vi "SSCP.vi"(0 "Config file path":path=path "F:/Projects/simple-system-control-protocol/simple-system-control-protocol/source/python/lp_em_cc2340r5_example.yml", 1 "Parameter name":string, 2 "Parameter value":string, 3 "Register name":string, 5 "Device Configuration":T1={"Device name"="default", "Device number"="0", "Serial Port"="COM9", "Serial baud rate"="115200", "Base Port"="3000", "Device Serial Number"="1", "Interface Timeout"="10000", "Interface Type"="SERIAL"}, 11 "error in (no error)":errorcluster, 12 "Command":T2) -> (4 "Parameter value":dbl, 15 "error out":errorcluster)   [LabVIEW 2020]
uses:
  commands.ctl
  typedefs/Device Configuration.ctl
  typedefs/Parameter Descriptor.ctl
  typedefs/Register Descriptor.ctl
  <vilib>/regexp/Match Regular Expression.xnode
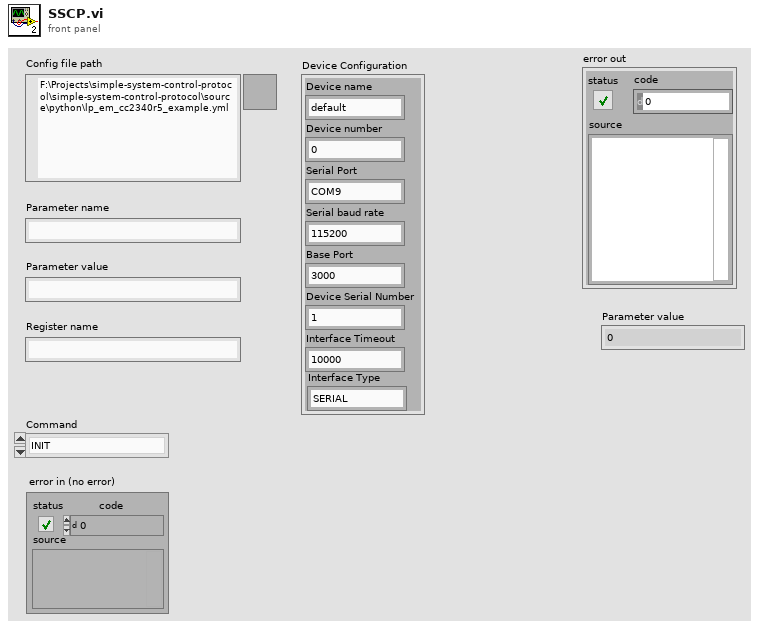
[diagram p1: front panel]
types:
  T1 = typedef "Device Configuration.ctl" = cluster{"Device name":string, "Device number":string, "Serial Port":string, "Serial baud rate":string, "Base Port":string, "Device Serial Number":string, "Interface Timeout":string, "Interface Type":string}
  T2 = typedef "commands.ctl" = enum16{"INIT", "CONFIGURE", "CONNECT", "GET_PARAMETER", "GET_PARAMETER_FROM_DEVICE", "SET_PARAMETER", "SET_PARAMETER_IN_DEVICE", "READ_REGISTER", "WRITE_REGISTER", "DISCONNECT"}
  T3 = typedef "Register Descriptor.ctl" = cluster{"Parameter Descriptors":T4[], "Register name":string, "Register number":i32}
  T4 = typedef "Parameter Descriptor.ctl" = cluster{"Register name":string, "Parameter name":string, "Register number":i32, "Parameter number":i32, "Start Bit":i32, "Bit Length":i32, "min":string, "max":string, "datatype":string}
  T5 = enum16{"Standard", "Buffered", "CRLF", "Immediate"}
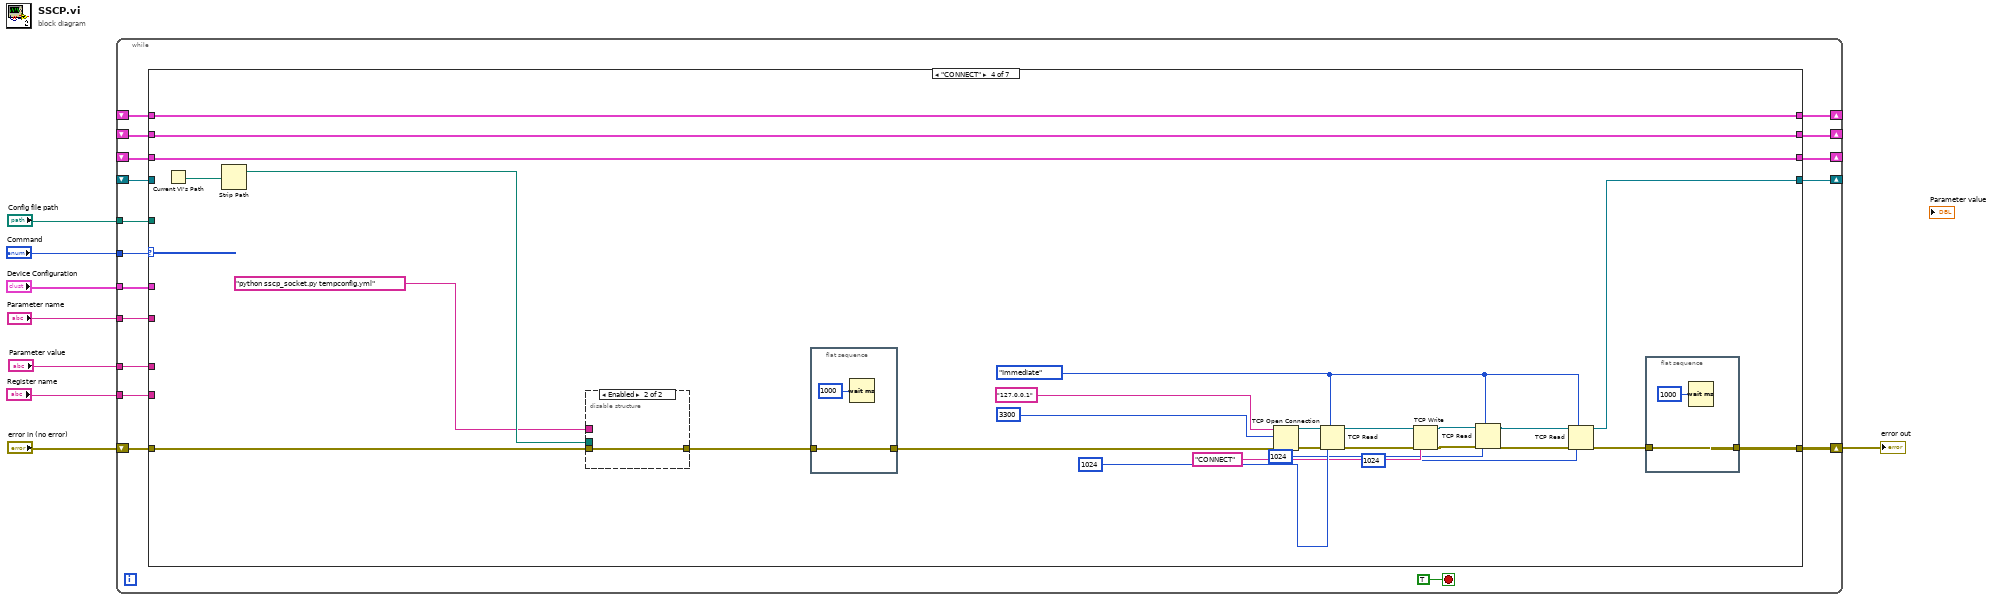
[diagram p0: block diagram]
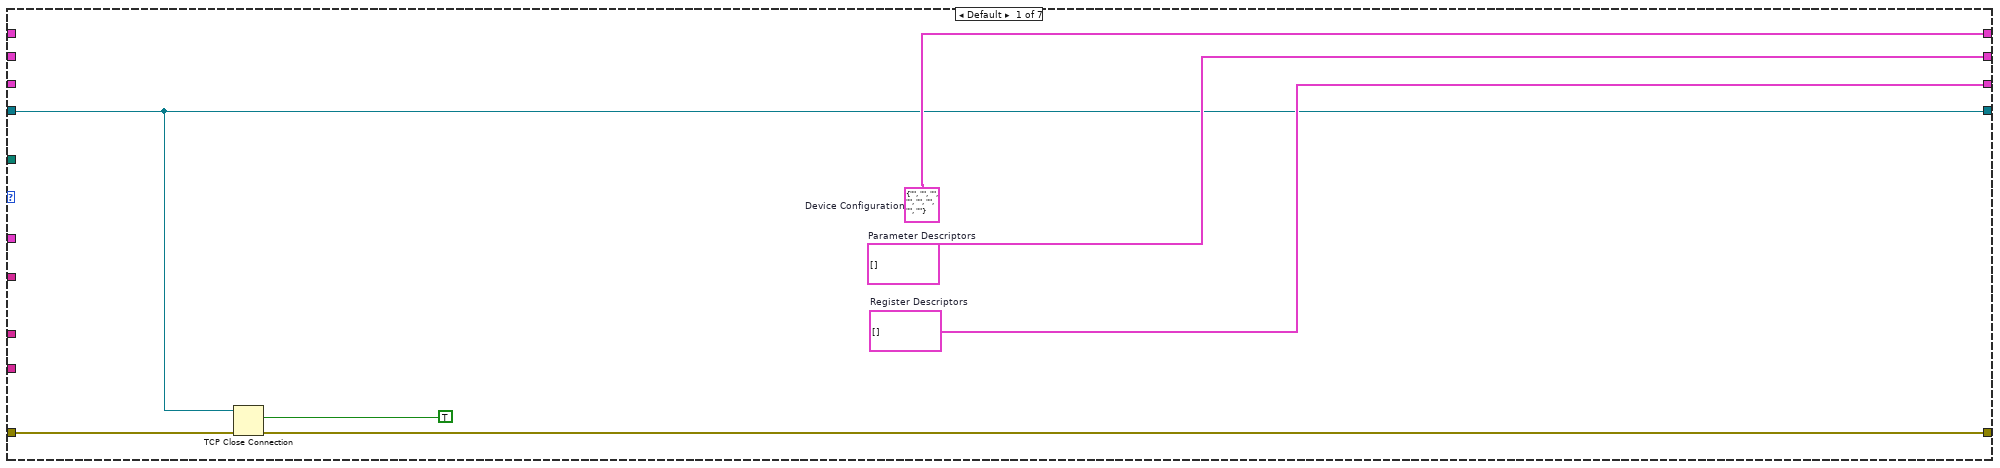
[diagram p2: hidden frame]
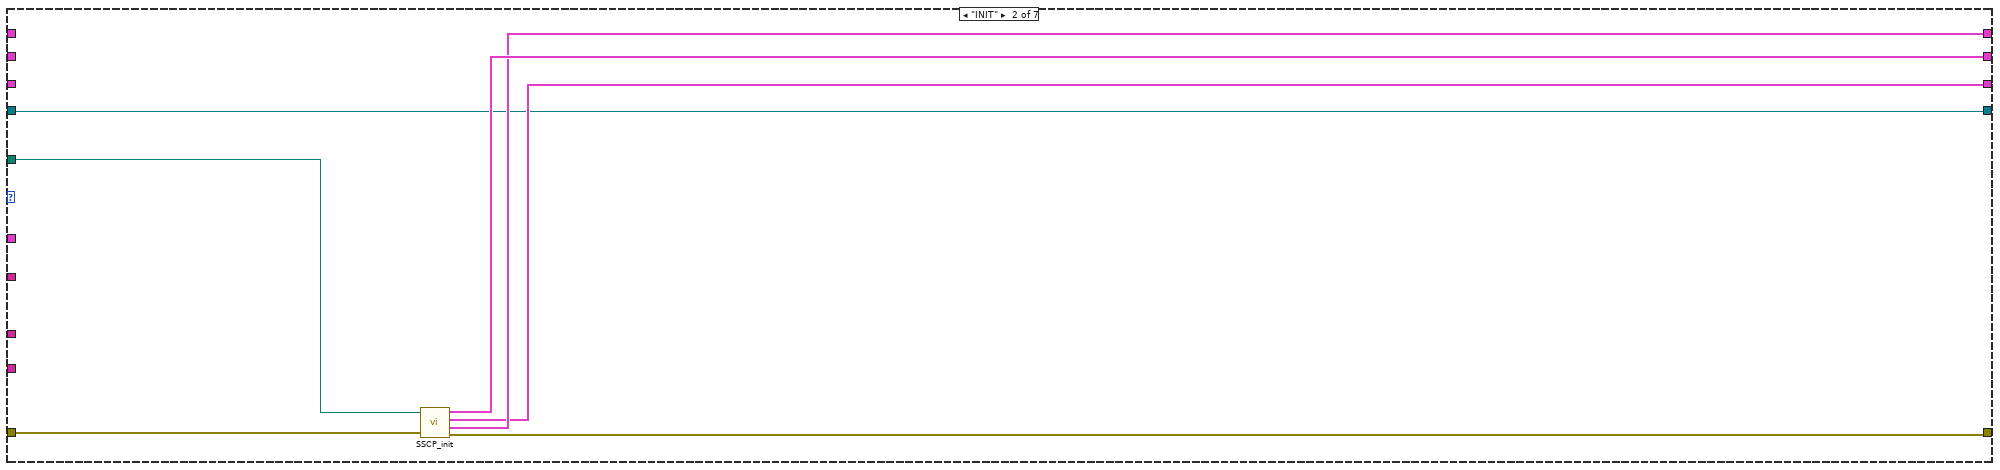
[diagram p3: hidden frame]
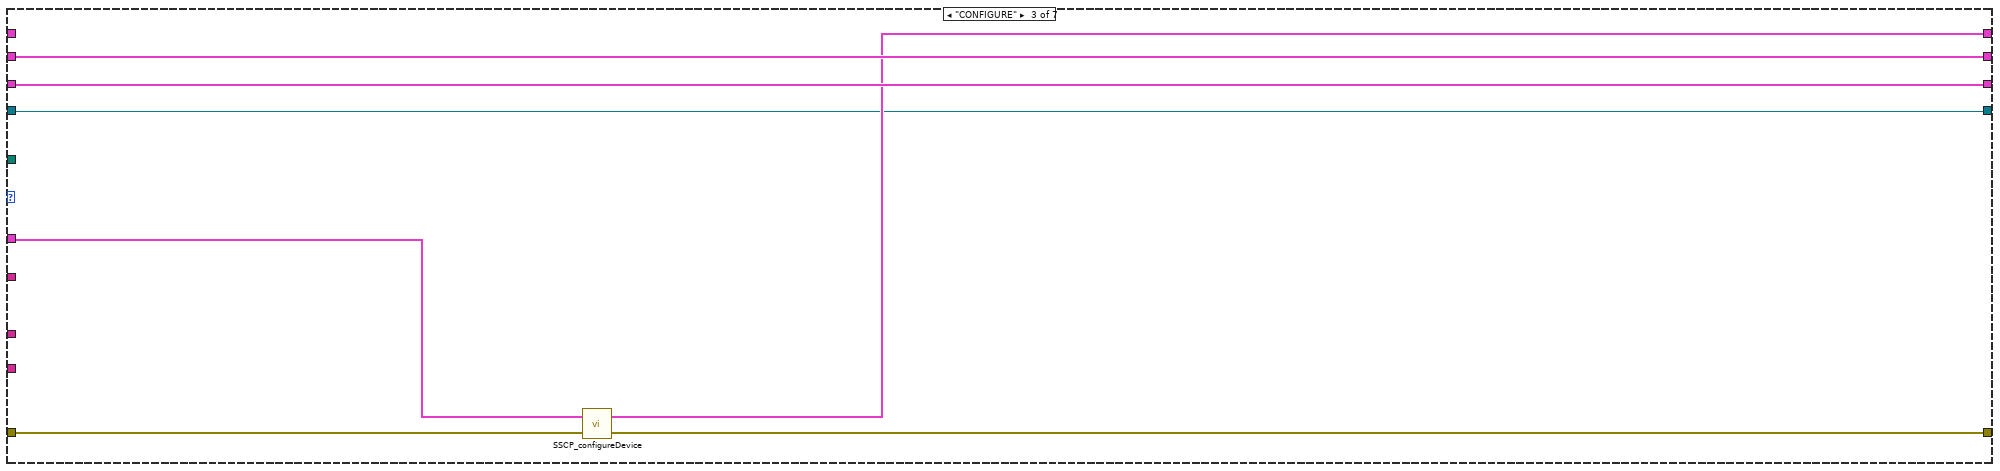
[diagram p4: hidden frame]
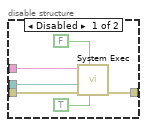
[diagram p5: hidden frame]
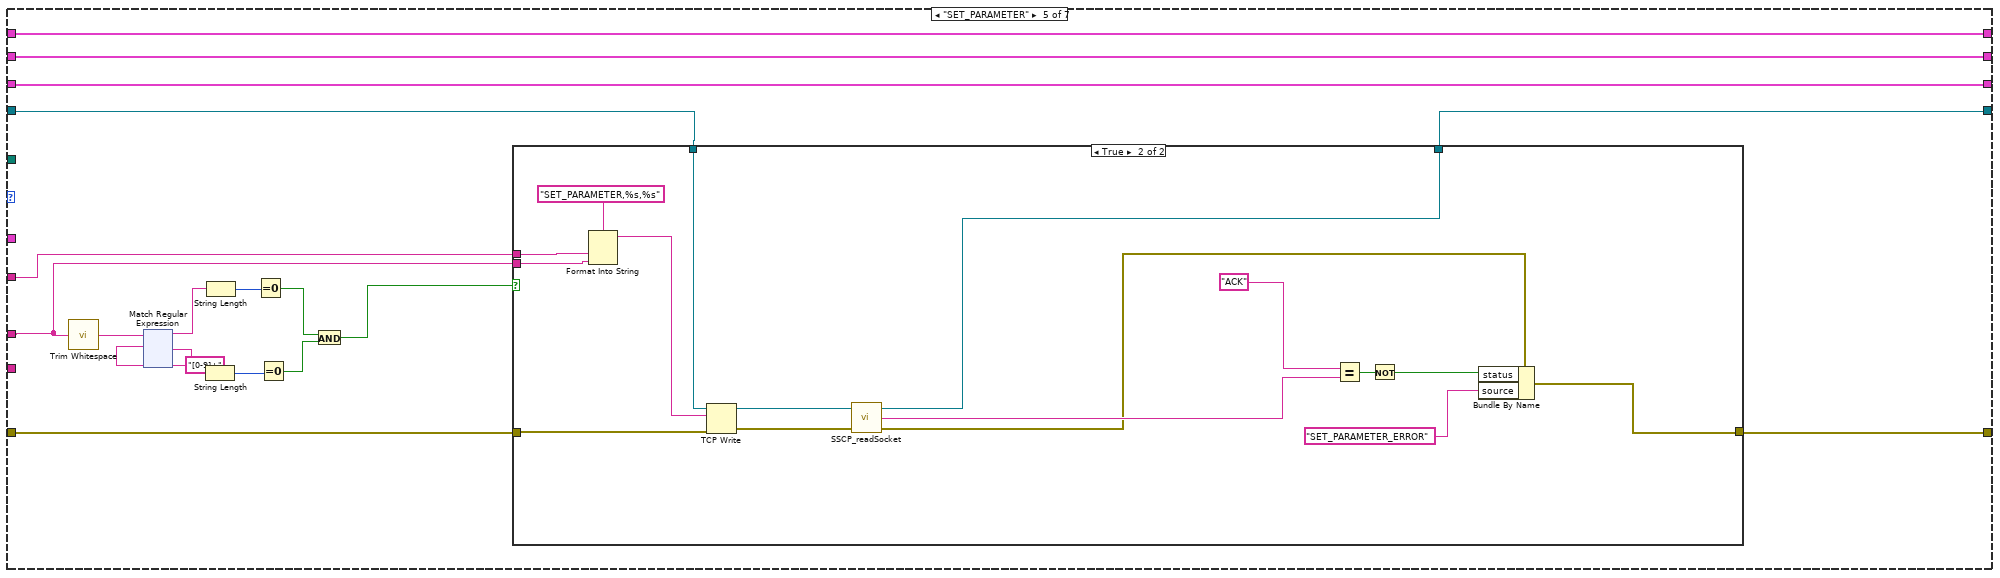
[diagram p6: hidden frame]
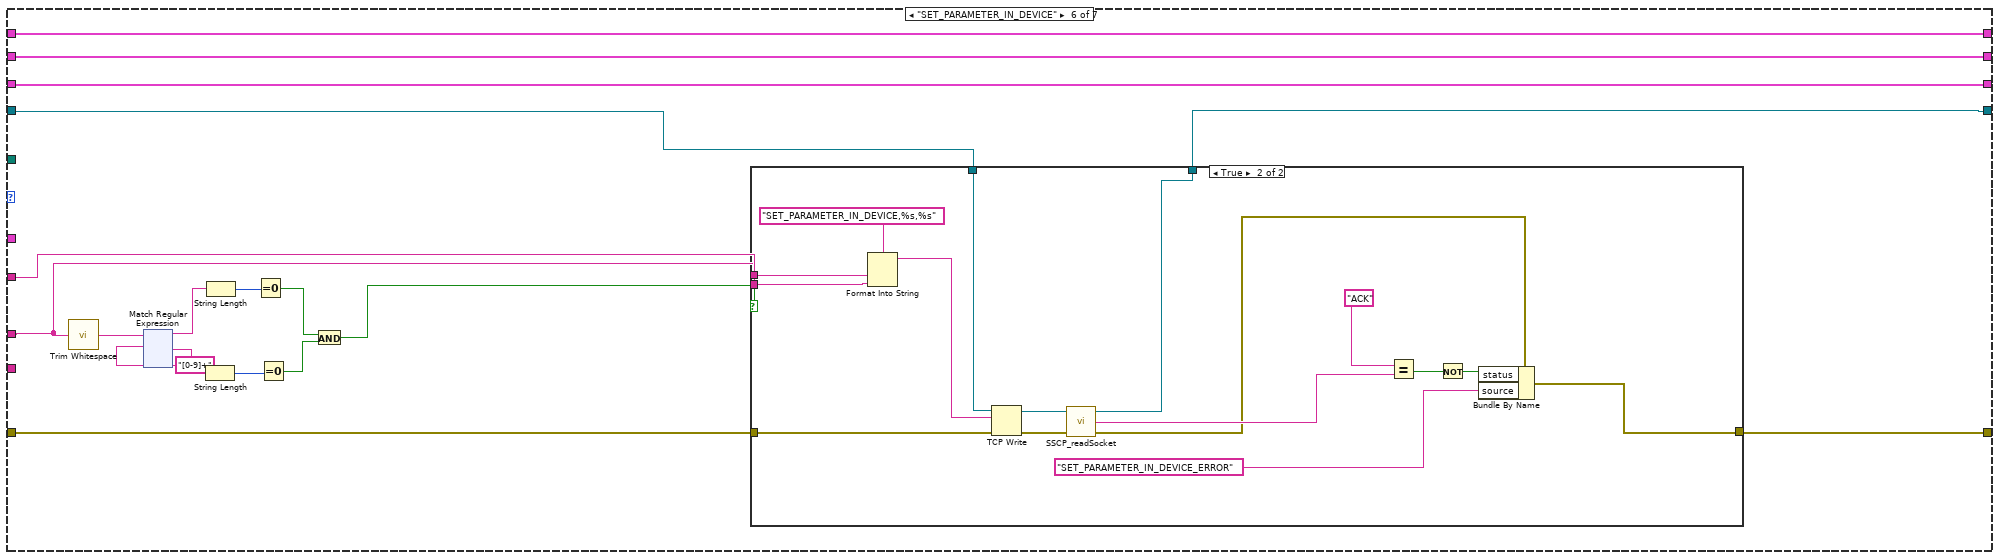
[diagram p8: hidden frame]
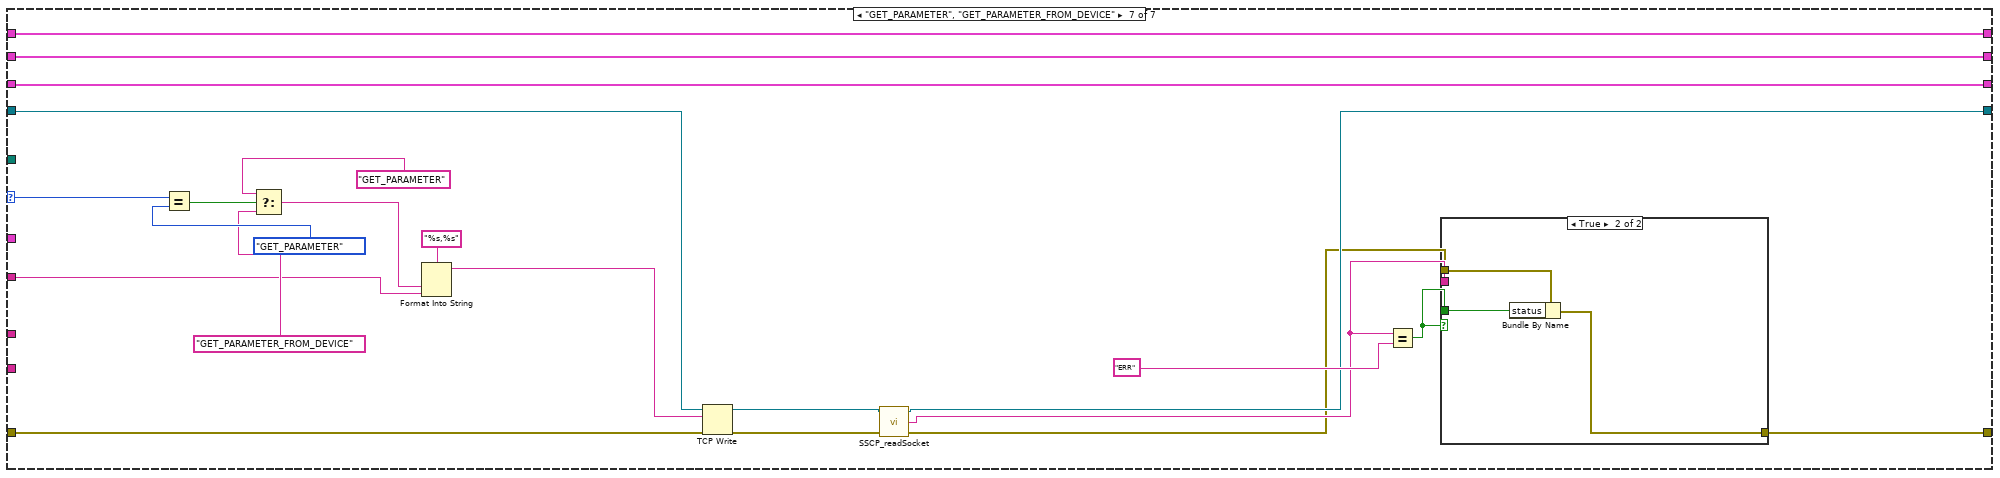
[diagram p10: hidden frame]
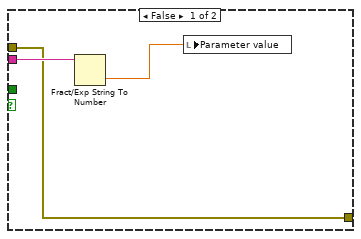
[diagram p11: hidden frame]
diagram:
  n1 = while {
    tunnel: "Command" -> [w25]
    tunnel: "Config file path" -> [w23]
    tunnel: "Device Configuration" -> [w22]
    tunnel: "Parameter name" -> [w21]
    tunnel: "Parameter value" -> [w20]
    tunnel: "Register name" -> [w19]
    shift-right: [w18] -> w1
    shift-left: "error in (no error)" -> [w24]
    shift-right: [w16] -> _
    shift-left: _ -> [w11]
    shift-right: [w15] -> _
    shift-left: _ -> [w13]
    shift-right: [w14] -> _
    shift-left: _ -> [w12]
    shift-right: [w10] -> _
    shift-left: _ -> [w9]
    stop <- TRUE stop-if-true
    n2 = case shown="\"CONNECT\"" w25 {
      selector: w25 -> [_ _ _ _ _ _ w406]
      tunnel: w24 -> [w29 w39 w44 w69 w99 w249 w398]
      tunnel: w23 -> [_ w38 _ _ _ _ _]
      tunnel: w22 -> [_ _ w43 _ _ _ _]
      tunnel: w21 -> [_ _ _ _ w89 w238 w399]
      tunnel: w20 -> [_ _ _ _ w87 w236 _]
      tunnel: w19 -> [_ _ _ _ _ _ _]
      tunnel: [w26 w37 w41 w48 w88 w237 w392] -> w18
      tunnel: [w32 w35 w42 w61 w102 w252 w395] -> w16
      tunnel: [w31 w36 w46 w73 w101 w251 w394] -> w15
      tunnel: [w30 w34 w45 w72 w100 w250 w393] -> w14
      tunnel: w13 -> [_ _ w46 w73 w101 w251 w394]
      tunnel: w12 -> [_ _ w45 w72 w100 w250 w393]
      tunnel: w11 -> [_ _ _ w61 w102 w252 w395]
      tunnel: [w28 w33 w40 w50 w86 w235 w387] -> w10
      tunnel: w9 -> [w28 w33 w40 _ w85 w248 w397]
      frame Default {
        w30 = T3[] []  # Register Descriptors
        w31 = T4[] []  # Parameter Descriptors
        w32 = T1 {"Device name"="", "Device number"="", "Serial Port"="", "Serial baud rate"="", "Base Port"="", "Device Serial Number"="", "Interface Timeout"="", "Interface Type"=""}  # Device Configuration
        n3 = TCP Close Connection(connection ID=w28, abort (F)=TRUE, error in (no error)=w29) -> (error out=w26:errorcluster)  [unwired: 1 out]
      }
      frame "INIT" {
        n4 = call "SSCP_init.vi"("config file"=w38, "error in (no error)"=w39) -> ("Parameter Descriptors"=w36:T4[], "Register Descriptors"=w34:T3[], "Device Configuration"=w35:T1, "error out"=w37:errorcluster)  [unwired: 1 in]
      }
      frame "CONFIGURE" {
        n5 = call "SSCP_configureDevice.vi"("error in (no error)"=w44, "Device Configuration in"=w43) -> ("error out"=w41:errorcluster, "Device Configuration out"=w42:T1)
      }
      frame "CONNECT" {
        w51 = T5."Immediate" ("mode (standard)")
        n6 = Current VI's Path() -> (path=w71:path)
        n7 = Strip Path(path=w71) -> (stripped path=w70:path)  [unwired: 1 out]
        n8 = disable-structure shown="Enabled" {
          disable-tunnel: w70 -> [w80 _]
          disable-tunnel: w69 -> [w78 w82]
          disable-tunnel: [w77 w82] -> w63
          disable-tunnel: "python sscp_socket.py tempconfig.yml" ("command line") -> [w76 _]
          frame Disabled {
            n9 = call <vilib>:"System Exec.vi"("run minimized? (F)"=TRUE, "wait until completion? (T)"=FALSE, "error in (no error)"=w78, "working directory"=w80, "command line"=w76) -> ("error out"=w77:errorcluster)  [unwired: 3 in, 3 out]
          }
          frame Enabled {
          }
        }
        n10 = flat-sequence {
          tunnel: w63 -> [w84]
          tunnel: [w84] -> w62
          frame #0 {
            n11 = Wait (ms)(milliseconds to wait=u32 1000) -> ()  [unwired: 1 out]
          }
        }
        n12 = TCP Open Connection(address="127.0.0.1", remote port or service name=u16 3300, error in (no error)=w62) -> (connection ID=w65:refnum<k5>, error out=w66:errorcluster)  [unwired: 2 in]
        n13 = TCP Read(connection ID=w65, bytes to read=1024, error in (no error)=w66, 7:w51) -> (connection ID out=w59:refnum<k5>, error out=w60:errorcluster)  [unwired: 1 in, 1 out]
        n14 = TCP Write(connection ID=w59, data in="CONNECT", error in (no error)=w60) -> (connection ID out=w56:refnum<k5>, error out=w57:errorcluster)  [unwired: 1 in, 1 out]
        n15 = TCP Read(connection ID=w56, bytes to read=1024, error in (no error)=w57, 7:w51) -> (connection ID out=w52:refnum<k5>, error out=w54:errorcluster)  [unwired: 1 in, 1 out]
        n16 = TCP Read(connection ID=w52, bytes to read=1024, error in (no error)=w54, 7:w51) -> (connection ID out=w50:refnum<k5>, error out=w49:errorcluster)  [unwired: 1 in, 1 out]
        n17 = flat-sequence {
          tunnel: w49 -> [w75]
          tunnel: [w75] -> w48
          frame #0 {
            n18 = Wait (ms)(milliseconds to wait=u32 1000) -> ()  [unwired: 1 out]
          }
        }
      }
      frame "SET_PARAMETER" {
        n19 = call <vilib>:"Trim Whitespace.vi"("string"=w87) -> ("trimmed string"=w98:string)  [unwired: 1 in]
        n20 = xnode "Match Regular Expression"("input string"=w98, "regular expression"="[0-9]+") -> ("before match"=w96:string, "after match"=w95:string)  [unwired: 4 in, 3 out]
        n21 = String Length(string=w95) -> (length=w93:i32)
        n22 = String Length(string=w96) -> (length=w94:i32)
        n23 = Equal To 0?(x=w94) -> (x = 0?=w92:bool)
        n24 = Equal To 0?(x=w93) -> (x = 0?=w91:bool)
        n25 = And(x=w92, y=w91) -> (x .and. y?=w90:bool)
        n26 = case shown="True" w90 {
          tunnel: w99 -> [w104 w120]
          tunnel: w85 -> [w103 w119]
          tunnel: w89 -> [_ w117]
          tunnel: [w104 w106] -> w88
          tunnel: w87 -> [_ w112]
          tunnel: [w103 w109] -> w86
          frame False {
          }
          frame True {
            n27 = Format Into String(format string="SET_PARAMETER,%s,%s", w117, w112) -> (resulting string=w116:string)  [unwired: 2 in, 1 out]
            n28 = TCP Write(connection ID=w119, data in=w116, error in (no error)=w120) -> (connection ID out=w111:refnum<k5>, error out=w110:errorcluster)  [unwired: 1 in, 1 out]
            n29 = call "SSCP_readSocket.vi"("error in"=w110, "connection in"=w111) -> ("error out"=w107:errorcluster, "payload"=w108:string, "connection out"=w109:refnum<k5>)  [unwired: 1 in]
            n30 = Equal?(x="ACK", y=w108) -> (x = y?=w114:bool)
            n31 = Not(x=w114) -> (.not. x?=w113:bool)
            n32 = Bundle By Name(cluster=w107, "status"=w113, "source"="SET_PARAMETER_ERROR") -> (w106:errorcluster)
          }
        }
      }
      frame "SET_PARAMETER_IN_DEVICE" {
        n33 = call <vilib>:"Trim Whitespace.vi"("string"=w236) -> ("trimmed string"=w247:string)  [unwired: 1 in]
        n34 = xnode "Match Regular Expression"("input string"=w247, "regular expression"="[0-9]+") -> ("before match"=w245:string, "after match"=w244:string)  [unwired: 4 in, 3 out]
        n35 = String Length(string=w244) -> (length=w242:i32)
        n36 = String Length(string=w245) -> (length=w243:i32)
        n37 = Equal To 0?(x=w243) -> (x = 0?=w241:bool)
        n38 = Equal To 0?(x=w242) -> (x = 0?=w240:bool)
        n39 = And(x=w241, y=w240) -> (x .and. y?=w239:bool)
        n40 = case shown="True" w239 {
          tunnel: w249 -> [w254 w270]
          tunnel: w248 -> [w253 w269]
          tunnel: w238 -> [_ w267]
          tunnel: [w254 w258] -> w237
          tunnel: w236 -> [_ w262]
          tunnel: [w253 w259] -> w235
          frame False {
          }
          frame True {
            n41 = Format Into String(format string="SET_PARAMETER_IN_DEVICE,%s,%s", w267, w262) -> (resulting string=w266:string)  [unwired: 2 in, 1 out]
            n42 = TCP Write(connection ID=w269, data in=w266, error in (no error)=w270) -> (connection ID out=w260:refnum<k5>, error out=w261:errorcluster)  [unwired: 1 in, 1 out]
            n43 = call "SSCP_readSocket.vi"("error in"=w261, "connection in"=w260) -> ("error out"=w255:errorcluster, "payload"=w256:string, "connection out"=w259:refnum<k5>)  [unwired: 1 in]
            n44 = Equal?(x="ACK", y=w256) -> (x = y?=w264:bool)
            n45 = Not(x=w264) -> (.not. x?=w263:bool)
            n46 = Bundle By Name(cluster=w255, "status"=w263, "source"="SET_PARAMETER_IN_DEVICE_ERROR") -> (w258:errorcluster)
          }
        }
      }
      frame "GET_PARAMETER", "GET_PARAMETER_FROM_DEVICE" {
        n47 = Equal?(x=w406, y=commands."GET_PARAMETER") -> (x = y?=w404:bool)
        n48 = Select(t="GET_PARAMETER" ("format string"), s=w404, f="GET_PARAMETER_FROM_DEVICE" ("format string")) -> (s? t:f=w400:string)
        n49 = Format Into String(format string="%s,%s", w400, w399) -> (resulting string=w396:string)  [unwired: 2 in, 1 out]
        n50 = TCP Write(connection ID=w397, data in=w396, error in (no error)=w398) -> (connection ID out=w389:refnum<k5>, error out=w388:errorcluster)  [unwired: 1 in, 1 out]
        n51 = call "SSCP_readSocket.vi"("error in"=w388, "connection in"=w389) -> ("error out"=w385:errorcluster, "payload"=w386:string, "connection out"=w387:refnum<k5>)  [unwired: 1 in]
        n52 = Equal?(x=w386, y="ERR") -> (x = y?=w391:bool)
        n53 = case shown="True" w391 {
          tunnel: w385 -> [w407 w412]
          tunnel: w391 -> [_ w411]
          tunnel: [w407 w410] -> w392
          tunnel: w386 -> [w409 _]
          frame False {
            n54 = Fract/Exp String To Number(string=w409) -> (number=w408:dbl)  [unwired: 3 in, 1 out]
            n55 = local write "Parameter value"(w408) -> ()
          }
          frame True {
            n56 = Bundle By Name(cluster=w412, "status"=w411) -> (w410:errorcluster)
          }
        }
      }
    }
  }
  "error out" <- w1
